vi "Start Streaming.vi"(5 "Max Sequential Frame-Errors (Default: -1)":i32=-1, 6 "Stream Acquisition Type (Default: Continuous)":T1, 7 "Additional Buffers (Default: 3)":u16=3, 8 "error in (no error)":errorcluster, 9 "Timeout (ms)":i32=10000, 11 "Camera in":refnum<class "Camera.lvclass">) -> (0 "error out":errorcluster, 3 "Camera":refnum<class "Camera.lvclass">)   [LabVIEW 2020, in "Camera.lvclass"]
uses:
  Camera.lvclass
  Camera.lvclass/Camera.ctl
  Event Type.ctl
  Stream User Events.ctl
  bin/gindustrialcam_32-1.dll
  Stream Acquisition Type.ctl
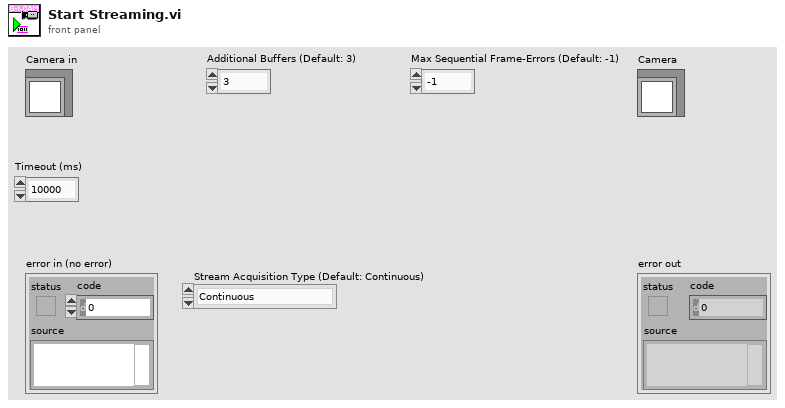
[diagram p1: front panel]
types:
  T1 = typedef "Camera.lvclass/Stream Acquisition Type.ctl" = enum8{"Continuous", "Fixed Frame Count"}
  T2 = typedef "Camera.lvclass/Stream User Events.ctl" = cluster{"Stopped":refnum<user-event>, "Errors":refnum<user-event>}
  T3 = typedef "Camera.lvclass/Streaming Registation.ctl" = cluster{"Streaming Events":refnum<event-registration>, "User Events":T2}
  T4 = typedef "Camera.lvclass/Event Type.ctl" = enum16{"Other", "Disconnect", "Stream Stop"}
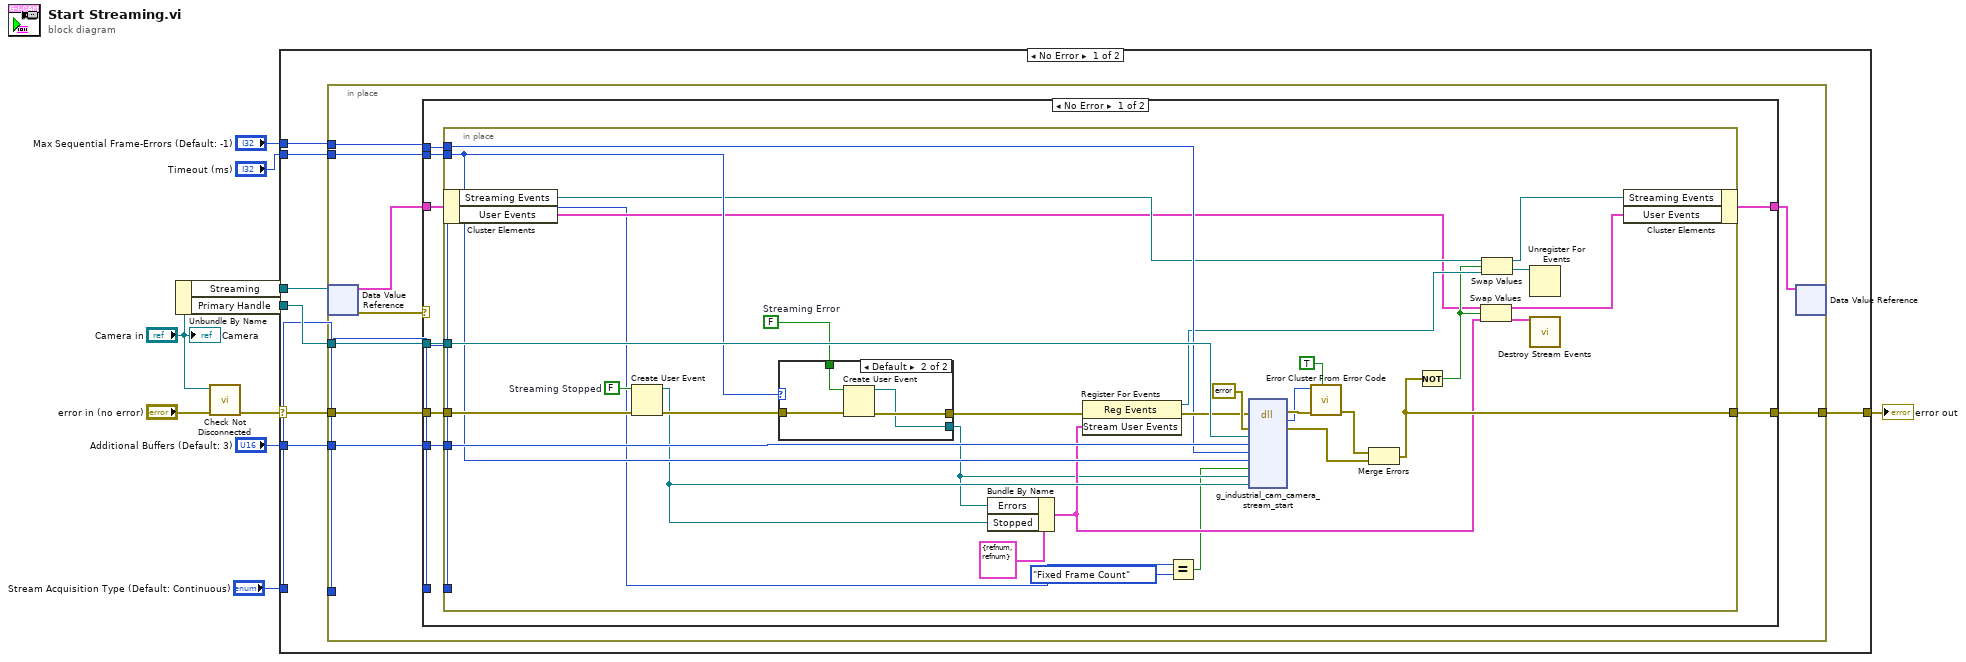
[diagram p0: block diagram]
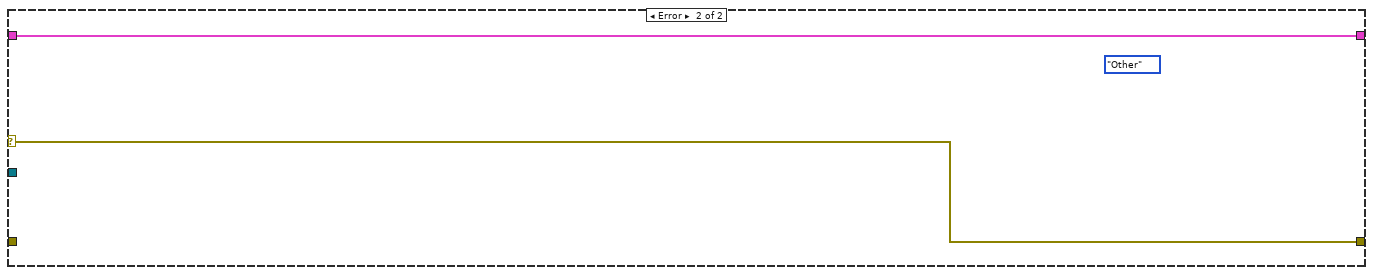
[diagram p3: hidden frame]
diagram:
  n1 = Unbundle By Name("Camera in") -> ("Streaming"=w6:refnum<data-value>, "Primary Handle"=w9:refnum<data-value>)
  n2 = call "Check Not Disconnected.vi"("error in (no error)"="error in (no error)", "Camera in"="Camera in") -> ("error out"=w7:errorcluster)  [unwired: 9 in]
  n3 = case shown="No Error" w7 {
    selector: w7 -> [w17 w77]
    tunnel: w9 -> [w18 _]
    tunnel: w6 -> [w16 _]
    tunnel: "Timeout (ms)" -> [w15 _]
    tunnel: [w13 w77] -> w4
    tunnel: "Additional Buffers (Default: 3)" -> [w14 _]
    tunnel: "Max Sequential Frame-Errors (Default: -1)" -> [w12 _]
    tunnel: "Stream Acquisition Type (Default: Continuous)" -> [w11 _]
    frame No Error {
      n4 = in-place {
        in-place-border: w18 -> [w28]
        in-place-border: w17 -> [w27]
        in-place-border: w15 -> [w24]
        in-place-border: w14 -> [w23]
        in-place-border: [w22] -> w13
        in-place-border: w12 -> [w20]
        in-place-border: w11 -> [w19]
        n5 = in-place-dvr #1(w16) -> (w25:T3, w26:errorcluster)
        n6 = case shown="No Error" w26 {
          selector: w26 -> [_ w75]
          tunnel: w28 -> [w37 _]
          tunnel: w27 -> [w36 _]
          tunnel: w25 -> [w35 w76]
          tunnel: w24 -> [w34 _]
          tunnel: w23 -> [w33 _]
          tunnel: [w30 w75] -> w22
          tunnel: [w32 w76] -> w21
          tunnel: w20 -> [w31 _]
          tunnel: w19 -> [w29 _]
          frame No Error {
            n7 = in-place {
              in-place-border: w37 -> [w63]
              in-place-border: w36 -> [w57]
              in-place-border: w34 -> [w54]
              in-place-border: w33 -> [w58]
              in-place-border: w31 -> [w55]
              in-place-border: [w51] -> w30
              in-place-border: w29 -> [w40]
              w59 = FALSE  # Streaming Error
              w62 = FALSE  # Streaming Stopped
              n8 = in-place-cluster #2(w35) -> ("Streaming Events"=w50:refnum<event-registration>, "User Events"=w45:T2)
              n9 = Create User Event(user event datatype=w62, error in=w57) -> (user event=w52:refnum<user-event>, error out=w61:errorcluster)
              n10 = case shown="Default" w54 {
                tunnel: w61 -> [w70 w74]
                tunnel: [w70 w73] -> w60
                tunnel: [_ w72] -> w41
                tunnel: w59 -> [_ w71]
                frame ..-1 {
                }
                frame Default {
                  n11 = Create User Event(user event datatype=w71, error in=w74) -> (user event=w72:refnum<user-event>, error out=w73:errorcluster)
                }
              }
              n12 = Bundle By Name(cluster=T2 {"Stopped"=refnum, "Errors"=refnum} ("Stream User Events"), "Errors"=w41, "Stopped"=w52) -> (w44:T2)
              n13 = register-events(error in=w60, w44) -> (reference out=w49:refnum<event-registration>, error out=w56:errorcluster)  [unwired: 1 in]
              n14 = Equal?(x=w40, y=Stream_Acquisition_Type."Fixed Frame Count") -> (x = y?=w38:bool)
              n15 = dll-call lib="C:/serenial/lib/g-industrial-camera/LabVIEW/g_industrial_cam/bin/gindustrialcam_*-1.*" fn="g_industrial_cam_camera_stream_start"(error in=w56, "err"=errorcluster {"status"=FALSE, "code"=0, "source"=""} ("error constant"), "cam_edvr"=w63, "additional_buffers"=w58, "max_errors"=w55, "timeout_ms"=w54, "use_frame_count"=w38, "streaming_started_event"=w41, "streaming_stopped_event"=w52) -> (error out=w69:errorcluster, "Mg_Error"=w68:i32, "err"=w66:errorcluster)  [unwired: 9 in, 1 out]
              n16 = call <vilib>:"Error Cluster From Error Code.vi"("show call chain? (False)"=TRUE, "error in (no error)"=w69, "error code (0)"=w68) -> ("error out"=w67:errorcluster)  [unwired: 6 in]
              n17 = Merge Errors(w67, w66) -> (w51:errorcluster)
              n18 = Not(x=w51) -> (.not. x?=w46:bool)
              n19 = Swap Values(12:w45, 13:w46, 14:w44) -> (1:w43:T2, 3:w42:T2)
              n20 = Swap Values(12:w50, 13:w46, 14:w49) -> (1:w48:refnum<event-registration>, 3:w47:refnum<event-registration>)
              n21 = Unregister For Events(event registration refnum=w47) -> ()  [unwired: 1 in, 1 out]
              n22 = call "Destroy Stream Events.vi"("Stream User Events"=w42) -> ()  [unwired: 10 in, 1 out]
              n23 = in-place-cluster #2("Streaming Events"=w48, "User Events"=w43) -> (w32:T3)
            }
          }
          frame Error {
            (unwired) Event_Type."Other" ("Event")
          }
        }
        n24 = in-place-dvr #1(w21) -> ()  [unwired: 2 out]
      }
    }
    frame Error {
    }
  }
  "error out" <- w4
  "Camera" <- "Camera in"
